vi "MCSGlobalVars.vi"() -> ()   [LabVIEW 2014]
uses:
  Controls/MCSselectTrigger.ctl
  Controls/MCSstate.ctl
panel:
  in  "errorCount":i8
  in  "MCSstate":T1
  in  "nOfBunches":i32
  in  "nOfBins":u32
  in  "delay(ticks)":u32
  in  "MCSSelectTrigger":T2
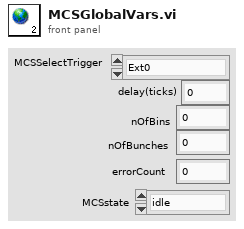
[diagram p1: front panel]
types:
  T1 = typedef "MCSstate.ctl" = enum16{"idle", "scanning", "done", "error"}
  T2 = typedef "MCSselectTrigger.ctl" = enum8{"Ext0", "Ext1", "Ext2", "Ext3", "Ext4", "Ext5", "Ext6", "Ext7", "Int0", "Int1", "Int2", "Int3", "Int4", "Int5", "Int6", "Int7"}
diagram:
